vi "Process.vi"(8 "Error In":errorcluster, 11 "CurrentResult In":refnum<class "CurrentResult.lvclass">) -> (0 "Error Out":errorcluster, 3 "CurrentResult Out":refnum<class "CurrentResult.lvclass">)   [LabVIEW 2020, in "CurrentResult.lvclass"]
uses:
  CurrentResult.lvclass
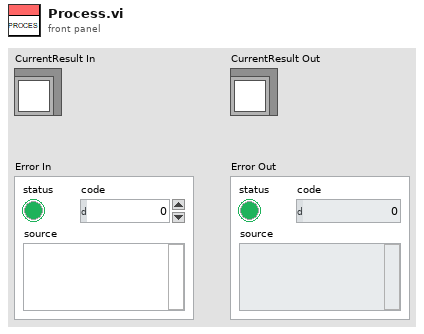
[diagram p1: front panel]
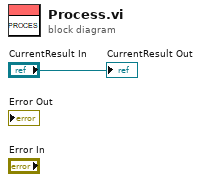
[diagram p0: block diagram]
diagram:
  "CurrentResult Out" <- "CurrentResult In"
